vi "Gif.CreatePicture.vi"(0 "image in":u32[][](array[colorbox]), 1 "Logical Screen Description":T2, 9 "offset":i32, 11 "error in (no error)":errorcluster) -> (4 "image out":picture, 10 "offset out":i32, 14 "graphic data":T1, 15 "error out":errorcluster)   [LabVIEW 2019]
uses:
  Gif.LogicalScreenDescriptior.ctl
  <vilib>/picture/picture.llb/imagedata.ctl
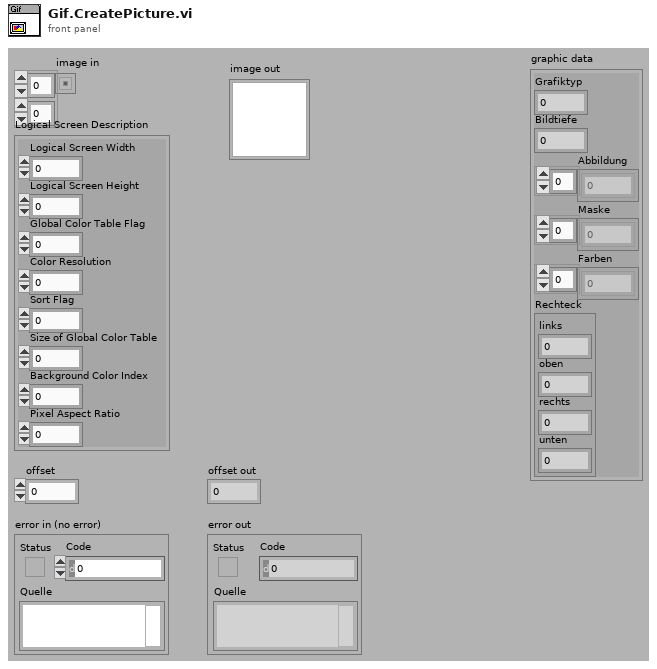
[diagram p1: front panel]
types:
  T1 = typedef "imagedata.ctl" = cluster{"image type":i32, "image depth":i32, "image":u8[], "mask":u8[], "colors":u32[], "Rectangle":cluster{"left":i16, "top":i16, "right":i16, "bottom":i16}}
  T2 = typedef "Gif.LogicalScreenDescriptior.ctl" = cluster{"Logical Screen Width":u16, "Logical Screen Height":u16, "Global Color Table Flag":u8, "Color Resolution":u8, "Sort Flag":u8, "Size of Global Color Table":u8, "Background Color Index":u8, "Pixel Aspect Ratio":u8}
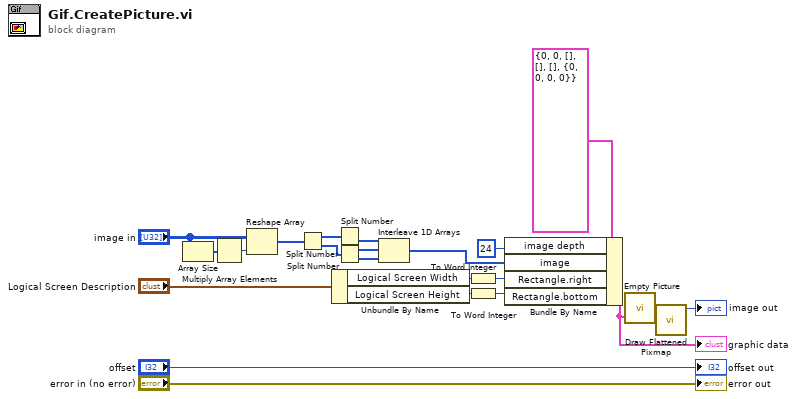
[diagram p0: block diagram]
diagram:
  n1 = Array Size(array="image in") -> (size(s)=w13:i32[])
  n2 = Multiply Array Elements(1:w13) -> (0:w12:i32)
  n3 = Reshape Array("image in", w12) -> (w6:u32[])
  n4 = Split Number(x=w6) -> (hi(x)=w5:u16[], lo(x)=w4:u16[])
  n5 = Unbundle By Name("Logical Screen Description") -> ("Logical Screen Width"=w16:u16, "Logical Screen Height"=w15:u16)
  n6 = Split Number(x=w5) -> (lo(x)=w3:u8[])  [unwired: 1 out]
  n7 = Split Number(x=w4) -> (hi(x)=w2:u8[], lo(x)=w1:u8[])
  n8 = Interleave 1D Arrays(w3, w2, w1) -> (w11:u8[])
  n9 = To Word Integer(number=w16) -> (16bit integer=w19:i16)
  n10 = To Word Integer(number=w15) -> (16bit integer=w18:i16)
  n11 = Bundle By Name(cluster=T1 {"image type"=0, "image depth"=0, "image"=[], "mask"=[], "colors"=[], "Rectangle"={"left"=0, "top"=0, "right"=0, "bottom"=0}} ("image data"), "image depth"=24, "image"=w11, "Rectangle.right"=w19, "Rectangle.bottom"=w18) -> (w21:T1)
  "graphic data" <- w21
  n12 = call "Empty Picture"() -> ("empty picture"=w10:picture)
  n13 = call <vilib>:"Draw Flattened Pixmap.vi"("image data"=w21, "picture"=w10) -> ("new picture"=→"image out":picture)  [unwired: 7 out]
  "error out" <- "error in (no error)"
  "offset out" <- "offset"
